vi "Vortex Klima schalten.vi"(0 "SOLL Temperatur":sgl, 2 "Delta T":sgl, 7 "IST Temperatur":sgl, 11 "error in (no error)":errorcluster caption="Fehler (Eingang, kein Fehler)") -> (4 "Ansteuerung":bool, 15 "error out":errorcluster caption="Fehler (Ausgang)")   [LabVIEW 2020, in "Allgemein.lvlib"]
uses:
  Allgemein.lvlib
panel:
  # "Ablaufinvariante Ausführung"
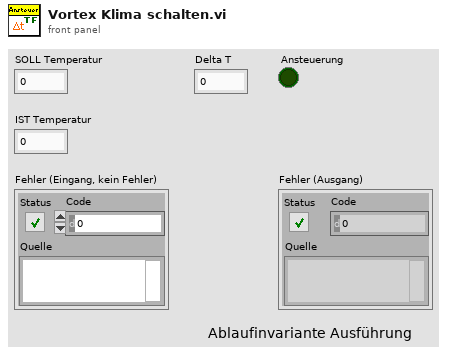
[diagram p1: front panel]
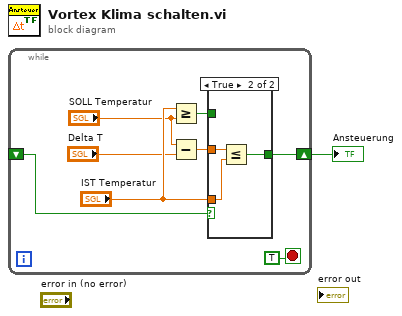
[diagram p0: block diagram]
diagram:
  n1 = while {
    shift-right: [w7] -> w1
    shift-left: _ -> [w9]
    stop <- TRUE stop-if-true
    n2 = Greater Or Equal?(x="IST Temperatur", y="SOLL Temperatur") -> (x >= y?=w8:bool)
    n3 = Subtract(x="SOLL Temperatur", y="Delta T") -> (x-y=w3:sgl)
    n4 = case shown="True" w9 {
      tunnel: w8 -> [w10 _]
      tunnel: [w10 w11] -> w7
      tunnel: "IST Temperatur" -> [_ w13]
      tunnel: w3 -> [_ w12]
      frame False {
      }
      frame True {
        n5 = Less Or Equal?(x=w12, y=w13) -> (x <= y?=w11:bool)
      }
    }
  }
  "Ansteuerung" <- w1
